vi "Check Decorator Actors.vi"(10 "Decorator Actors":refnum<class "Actor.lvclass">[](array[class])) -> (2 "Error":errorcluster)   [LabVIEW 2025, in "jettl.lvlib"]
uses:
  jettl.lvlib
  Actor/Actor.lvclass
  Error/Error.lvlib
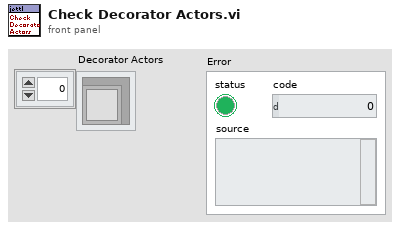
[diagram p1: front panel]
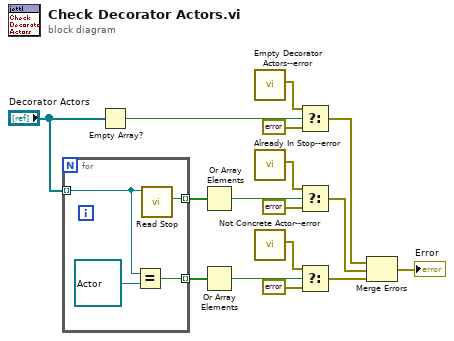
[diagram p0: block diagram]
diagram:
  n1 = for {
    tunnel: "Decorator Actors" -> [w18] mode=indexing
    tunnel: [w20] -> w11 mode=indexing
    tunnel: [w17] -> w7 mode=indexing
    n2 = Equal?(x=w18, y=refnum<class "Actor.lvclass"> refnum ("jettl.lvlib:Actor.lvclass")) -> (x = y?=w17:bool)
    n3 = call-dynamic "Read Stop.vi"("Actor in"=w18) -> ("Stop"=w20:bool)  [unwired: 10 in]
  }
  n4 = Empty Array?(array="Decorator Actors") -> (empty?=w14:bool)
  n5 = Or Array Elements(Boolean array=w11) -> (logical OR=w9:bool)
  n6 = Or Array Elements(Boolean array=w7) -> (logical OR=w4:bool)
  n7 = call "Empty Decorator Actors--error.vi"() -> ("Error"=w1:errorcluster)  [unwired: 11 in]
  n8 = call "Already In Stop--error.vi"() -> ("Error"=w6:errorcluster)  [unwired: 11 in]
  n9 = call "Not Concrete Actor--error.vi"() -> ("Error"=w3:errorcluster)  [unwired: 11 in]
  n10 = Select(t=w1, s=w14, f=errorcluster {"status"=FALSE, "code"=0, "source"=""}) -> (s? t:f=w13:errorcluster)
  n11 = Select(t=w6, s=w9, f=errorcluster {"status"=FALSE, "code"=0, "source"=""}) -> (s? t:f=w8:errorcluster)
  n12 = Select(t=w3, s=w4, f=errorcluster {"status"=FALSE, "code"=0, "source"=""}) -> (s? t:f=w2:errorcluster)
  n13 = Merge Errors(w13, w8, w2) -> (→"Error":errorcluster)
